vi "Fading_Out_VI.vi"(0 "Input Array":dbl[](array[numeric]), 7 "Fading length":dbl=400.0, 9 "Fading Index":i32, 11 "error in (no error)":errorcluster) -> (6 "Faded Array":dbl[](array[numeric]), 15 "error out":errorcluster)   [LabVIEW 2014]
doc: "VI zum Ausfaden eines Signals ab dem Fading Index über eine benutzerdefinierbare Länge (Fading length) [Standardwert: 400 samples]"
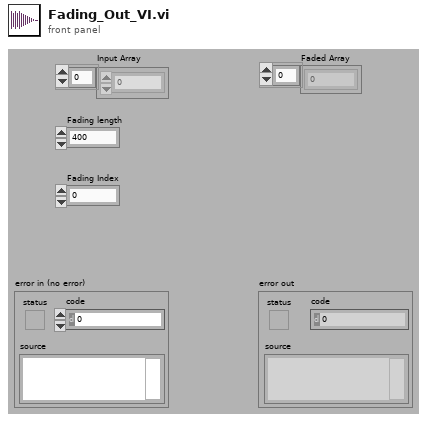
[diagram p1: front panel]
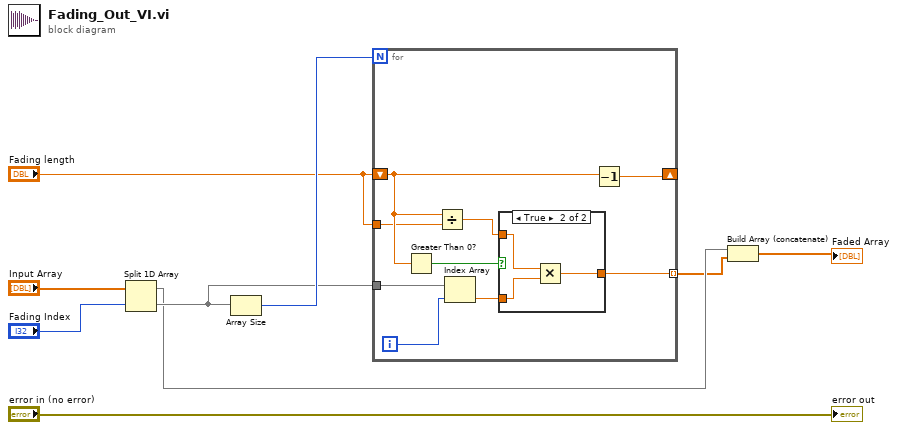
[diagram p0: block diagram]
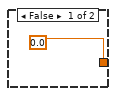
[diagram p2: hidden frame]
diagram:
  n1 = Split 1D Array(array="Input Array", index="Fading Index") -> (first subarray=w7:dbl[], second subarray=w8:dbl[])
  n2 = Array Size(array=w8) -> (size(s)=w9:i32)
  n3 = for {
    N: w9 -> [_]
    shift-right: [w16] -> _
    shift-left: "Fading length" -> [w12]
    tunnel: w8 -> [w17]
    tunnel: [w14] -> w4 mode=indexing
    tunnel: "Fading length" -> [w10]
    i -> [w18]
    n4 = Greater Than 0?(x=w12) -> (x > 0?=w11:bool)
    n5 = Divide(x=w12, y=w10) -> (x/y=w13:dbl)
    n6 = Index Array(array=w17, index=w18) -> (element=w15:dbl)
    n7 = case shown="True" w11 {
      tunnel: w13 -> [_ w22]
      tunnel: w15 -> [_ w21]
      tunnel: [0.0 w20] -> w14
      frame False {
      }
      frame True {
        n8 = Multiply(x=w22, y=w21) -> (x*y=w20:dbl)
      }
    }
    n9 = Decrement(x=w12) -> (x-1=w16:dbl)
  }
  n10 = Build Array (concatenate)(w7, w4) -> (→"Faded Array":dbl[])
  "error out" <- "error in (no error)"
